vi "PPAS-simulation-driverstation-comm.vi"(8 "error in (no error)":errorcluster, 11 "Occurrence Refnum":refnum<k4>) -> (0 "error out":errorcluster)   [LabVIEW 2019]
panel:
  out "cnx time":u32
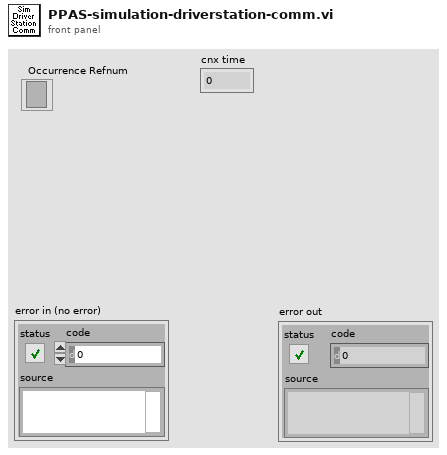
[diagram p1: front panel]
types:
  T1 = typedef "WPI_DriverStationRobotMode2.ctl" = enum16{"Autonomous Disabled", "Autonomous Enabled", "Teleop Disabled", "Teleop Enabled", "Disconnected", "Finish", "Test Disabled", "Test Enabled", "Emergency Stopped"}
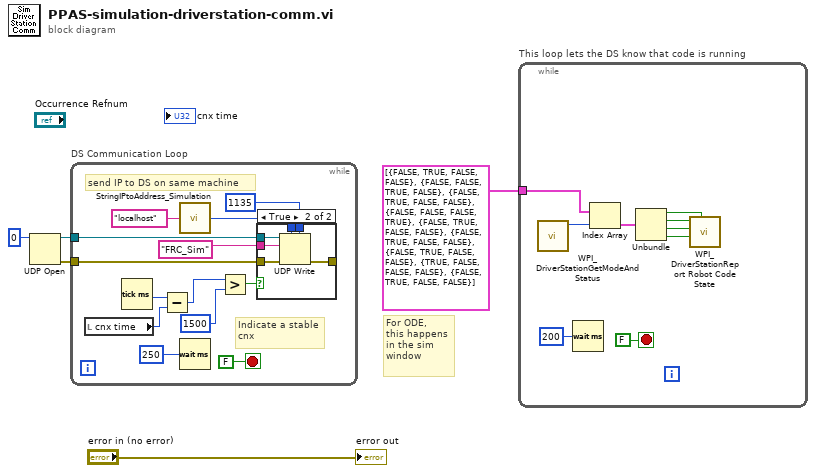
[diagram p0: block diagram]
diagram:
  # "For ODE,\nthis happens\nin the sim\nwindow"
  n1 = UDP Open(11:u16 0 ("port")) -> (port=w5:refnum<k16>, 0:w4:errorcluster)  [unwired: 4 in, 1 out]
  n2 = while "DS Communication Loop" {
    tunnel: w5 -> [w17]
    tunnel: w4 -> [w18]
    stop <- FALSE stop-if-true
    # "Indicate a stable\ncnx"
    # "send IP to DS on same machine"
    n3 = local read "cnx time"() -> (w10:u32)
    n4 = Tick Count (ms)() -> (millisecond timer value=w9:u32)
    n5 = Subtract(x=w9, y=w10) -> (x-y=w8:u32)
    n6 = call <vilib>:"StringIPtoAddress_Simulation.vi"("string IP"="localhost" ("DS IP 2")) -> ("address"=w14:u32)  [unwired: 14 in]
    n7 = Wait (ms)(milliseconds to wait=u32 250) -> ()  [unwired: 1 out]
    n8 = Greater?(x=w8, y=u32 1500 ("milliseconds to wait")) -> (0:w6:bool)
    n9 = case shown="True" w6 {
      tunnel: w18 -> [_ w24]
      tunnel: w17 -> [_ w23]
      tunnel: "FRC_Sim" ("data in") -> [_ w22]
      tunnel: w14 -> [_ w21]
      tunnel: [_ w20] -> _
      tunnel: u16 1135 ("port") -> [_ w19]
      frame False {
      }
      frame True {
        n10 = UDP Write(address=w21, port or service name=w19, connection ID=w23, data in=w22, 8:w24) -> (error out=w20:errorcluster)  [unwired: 1 in, 1 out]
      }
    }
  }
  n11 = while "This loop lets the DS know that code is running" {
    tunnel: cluster{bool, bool, bool, bool}[] [{FALSE, TRUE, FALSE, FALSE}, {FALSE, FALSE, TRUE, FALSE}, {FALSE, TRUE, FALSE, FALSE}, {FALSE, FALSE, FALSE, TRUE}, {FALSE, TRUE, FALSE, FALSE}, {FALSE, TRUE, FALSE, FALSE}, {FALSE, TRUE, FALSE, FALSE}, {TRUE, FALSE, FALSE, FALSE}, {FALSE, TRUE, FALSE, FALSE}] -> [w32]
    stop <- FALSE stop-if-true
    n12 = call <vilib>:"WPI_DriverStationGetModeAndStatus.vi"() -> ("Robot Mode"=w26:T1)  [unwired: 10 in, 1 out]
    n13 = Wait (ms)(milliseconds to wait=u32 200) -> ()  [unwired: 1 out]
    n14 = Index Array(array=w32, index=w26) -> (element=w27:cluster{bool, bool, bool, bool})
    n15 = Unbundle(w27) -> (w33:bool, w25:bool, w30:bool, w29:bool)
    n16 = call <vilib>:"WPI_DriverStationReport Robot Code State.vi"("Test"=w33, "TeleOp"=w29, "Autonomous"=w30, "Disabled"=w25) -> ()  [unwired: 7 in, 1 out]
  }
  "error out" <- "error in (no error)"
